vi "instance count allowed.vi"(8 "error in":errorcluster, 11 "Temperature Chamber Model configuration in":refnum<class "Temperature Chamber Model configuration.lvclass">) -> (0 "error out":errorcluster, 2 "instances allowed":i32, 3 "Temperature Chamber Model configuration out":refnum<class "Temperature Chamber Model configuration.lvclass">)   [LabVIEW 2015, in "Temperature Chamber Model configuration.lvclass"]
uses:
  Temperature Chamber Model configuration.lvclass
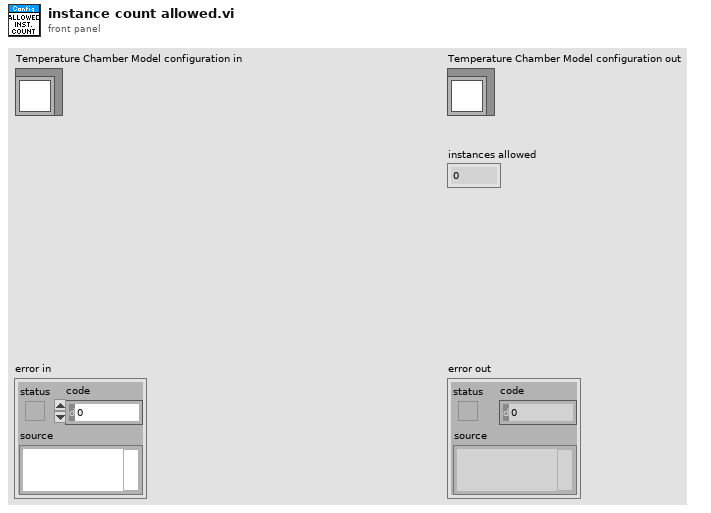
[diagram p1: front panel]
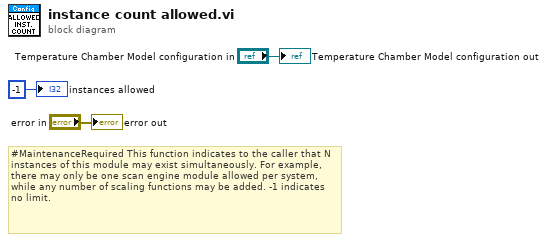
[diagram p0: block diagram]
diagram:
  # "#MaintenanceRequired This function indicates to the caller that N instances of this module may exist simultaneously. For example, there may only be one scan engine module allowed per system, while any number of scaling functions may be added. -1 indicates no limit."
  "error out" <- "error in"
  "Temperature Chamber Model configuration out" <- "Temperature Chamber Model configuration in"
  "instances allowed" <- -1 ("instances allowed")
